vi "CIE2T-Find Optimal Attenuation.vi"(0 "Acoustic System ID":string, 5 "Probe mic gain (dB)":dbl, 7 "Nominal Max SPL":dbl[](array[numeric]), 9 "DP Freqs":T1, 11 "error in (no error)":errorcluster) -> (8 "Attenuation (dB)":dbl[](array[numeric]), 15 "error out":errorcluster)   [LabVIEW 2020]
uses:
  cfts/LV Source/DPOAE VIs/Typedefs/DP-Freqs.ctl
  Utility VIs/Math VIs/interp1 (1D).vi
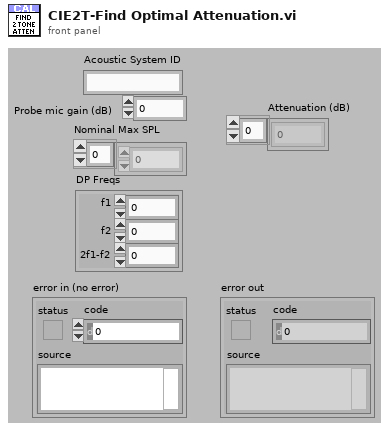
[diagram p1: front panel]
types:
  T1 = typedef "DP-Freqs.ctl" = cluster{"f1":dbl, "f2":dbl, "2f1-f2":dbl}
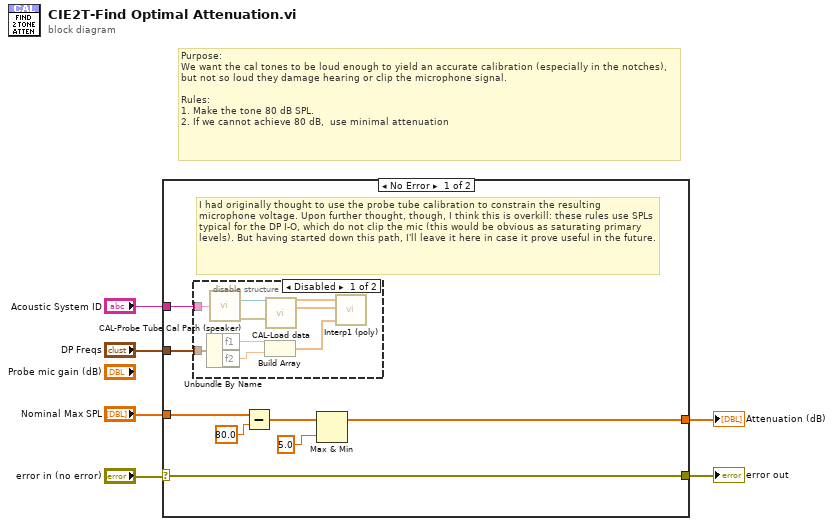
[diagram p0: block diagram]
diagram:
  # "Purpose: \nWe want the cal tones to be loud enough to yield an accurate calibration (especially in the notches), but not so loud they damage hearing or clip the microphone signal.\n\nRules: \n1. Make the tone 80 dB SPL.\n2. If we cannot achieve 80 dB,  use minimal attenuation"
  n1 = case shown="No Error" "error in (no error)" {
    selector: "error in (no error)" -> [w14 w24]
    tunnel: [w14 w24] -> w5
    tunnel: "Acoustic System ID" -> [w13 _]
    tunnel: "DP Freqs" -> [w12 _]
    tunnel: "Nominal Max SPL" -> [w11 _]
    tunnel: [w7 _] -> w1
    frame No Error {
      # "I had originally thought to use the probe tube calibration to constrain the resulting microphone voltage. Upon further thought, though, I think this is overkill: these rules use SPLs typical for the DP I-O, which do not clip the mic (this would be obvious as saturating primary levels). But having started down this path, I'll leave it here in case it prove useful in the future."
      n2 = disable-structure shown="Disabled" {
        disable-tunnel: w13 -> [w23 _]
        disable-tunnel: w12 -> [w20 _]
        frame Disabled {
          n3 = Unbundle By Name(w20) -> ("f1"=w19:dbl, "f2"=w18:dbl)
          n4 = call "CAL-Probe Tube Cal Path (speaker).vi"("Right"=w23) -> ("Probe Tube Cal Path"=w22:path, "error out"=w21:errorcluster)  [unwired: 13 in]
          n5 = Build Array(w19, w18) -> (w15:dbl[])
          n6 = call "CAL-Load data.vi"("user path"=w22, "error in (no error)"=w21) -> ("Frequency (Hz)"=w17:dbl[], "Mag"=w16:dbl[])  [unwired: 6 in, 6 out]
          n7 = call-poly "Interp1 (poly).vi"("U"=w15, "Y"=w16, "X"=w17) -> ()  [unwired: 1 out]
        }
        frame Enabled {
        }
      }
      n8 = Subtract(x=w11, y=80.0) -> (x-y=w9:dbl[])
      n9 = Max & Min(x=w9, y=5.0) -> (max(x,y)=w7:dbl[])  [unwired: 1 out]
    }
    frame Error {
    }
  }
  "error out" <- w5
  "Attenuation (dB)" <- w1
